vi "VeriStand Framework.Read.vi"(8 "error in (no error)":errorcluster, 10 "Data Ref":T1, 11 "VeriStand DSF in":refnum<class "VeriStand DSF.Framework.lvclass">) -> (0 "error out":errorcluster, 3 "VeriStand DSF out":refnum<class "VeriStand DSF.Framework.lvclass">)   [LabVIEW 2017, in "Data Sharing Framework Engine.lvlib" / "VeriStand DSF.Framework.lvclass"]
uses:
  VeriStand DSF.Framework.lvclass
  <vilib>/NI Veristand/Custom Device API/Data Table Ref.ctl
  DSF Core/Built/PharLap x86/Engine/c/DSF.Engine.lvlibp/Engine/Classes/Framework/DSF.Engine.Framework.lvclass
  C:/Git/DSF/DSF Core/Built/Windows/Engine/DSF.Engine.lvlibp/Engine/Classes/Framework/DSF.Engine.Framework.lvclass
  <vilib>/NI Veristand/Custom Device API/Custom Device API.lvlib
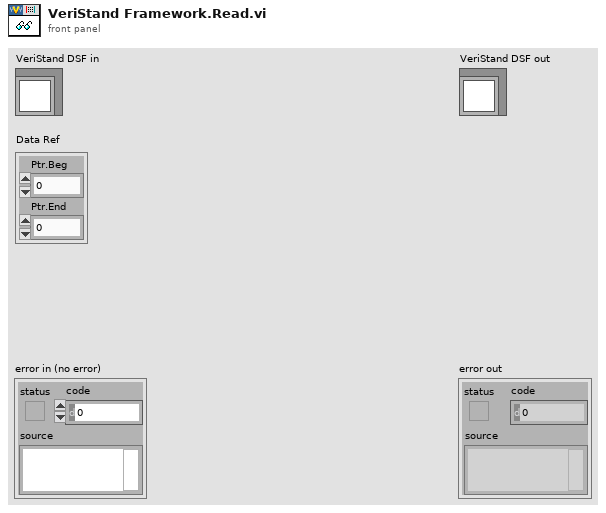
[diagram p1: front panel]
types:
  T1 = typedef "Custom Device API.lvlib/Data Table Ref.ctl" = cluster{"Ptr.Beg":u64, "Ptr.End":u64}
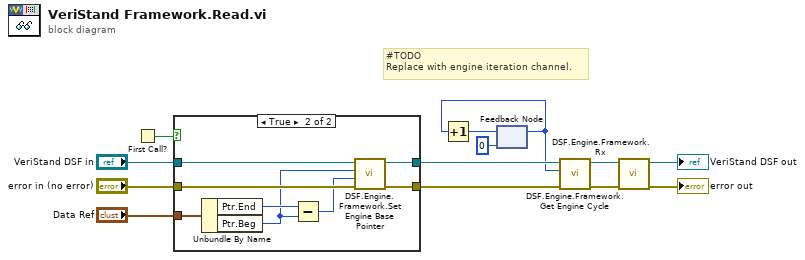
[diagram p0: block diagram]
diagram:
  # "#TODO\nReplace with engine iteration channel."
  n1 = First Call?() -> (First Call?: T/F=w7:bool)
  n2 = case shown="True" w7 {
    tunnel: "VeriStand DSF in" -> [w15 w19]
    tunnel: "error in (no error)" -> [w14 w18]
    tunnel: [w15 w21] -> w4
    tunnel: [w14 w20] -> w2
    tunnel: "Data Ref" -> [_ w23]
    frame False {
    }
    frame True {
      n3 = Unbundle By Name(w23) -> ("Ptr.End"=w22:u64, "Ptr.Beg"=w16:u64)
      n4 = Subtract(x=w22, y=w16) -> (x-y=w17:u64)
      n5 = call "DSF.Engine.Framework.Set Engine Base Pointer.vi"("error in (no error)"=w18, "engine size"=w17, "engine base address"=w16, "Framework in"=w19) -> ("error out"=w20:errorcluster, "Framework out"=w21:refnum<class "VeriStand DSF.Framework.lvclass">)  [unwired: 6 in]
    }
  }
  n6 = feedback #1(u64 0 ("iteration")) -> (w3:u64)
  n7 = Increment(x=w3) -> (x+1=w8:u64)
  n8 = feedback-in #1(w8) -> ()
  n9 = call "DSF.Engine.Framework.Get Engine Cycle.vi"("error in (no error)"=w2, "iteration"=w3, "Framework in"=w4) -> ("error out"=w11:errorcluster, "Framework out"=w13:refnum<class "VeriStand DSF.Framework.lvclass">)  [unwired: 7 in]
  n10 = call "DSF.Engine.Framework.Rx.vi"("error in (no error)"=w11, "Framework in"=w13) -> ("error out"=→"error out":errorcluster, "Framework out"=→"VeriStand DSF out":refnum<class "VeriStand DSF.Framework.lvclass">)  [unwired: 8 in]
